vi "negative floating point interpretation.vi"() -> ()   [LabVIEW 2019]
panel:
  in  "Scaling":dbl=10000000000.0 format="%#_13g"
  out "data":string="_ÿ¼ê"
  out "Numeric":dbl=-0.0356712609 format="%#_13g"
  in  "byte order (0:big-endian, network order)":T1(ring)=enum."little-endian"
  in  "the buffer that is read to be interpreted":string="\u0002\u0003\u0004_ÿ¼ê\u001aX"
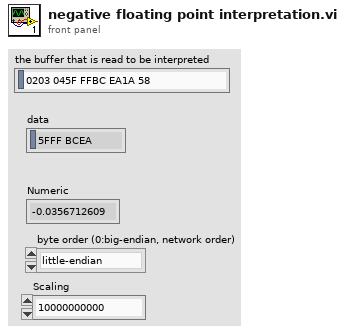
[diagram p1: front panel]
types:
  T1 = enum16{"big-endian, network order", "native, host order", "little-endian"}
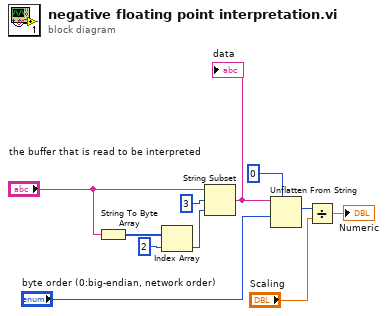
[diagram p0: block diagram]
diagram:
  n1 = String To Byte Array(string="the buffer that is read to be interpreted") -> (unsigned byte array=w10:u8[])
  n2 = Index Array(array=w10, index=2) -> (element=w6:u8)
  n3 = String Subset(string="the buffer that is read to be interpreted", offset (0)=3, length (rest)=w6) -> (substring=w5:string)
  "data" <- w5
  n4 = Unflatten From String(type=0, binary string=w5, byte order (0:big-endian, network order)="byte order (0:big-endian, network order)") -> (value=w2:i32)  [unwired: 2 in, 2 out]
  n5 = Divide(x=w2, y="Scaling") -> (x/y=→"Numeric":dbl)
